vi "RSZVB Trace Response Data All Data.vi"(8 "error in (no error)":errorcluster {"code" format="%.0x"}, 9 "Data Format (0)":i32(ring) items=["Unformatted", "Formatted", "Unformatted With Trace Mathematics"], 10 "Channel (Trace) (1)":i32=1, 11 "VISA session":refnum<visa-resource-name>) -> (0 "error out":errorcluster {"code" format="%.0x"}, 3 "dup VISA session":refnum<visa-resource-name>, 5 "Trace Data":dbl[](array[numeric]) format="%^.3e")   [LabVIEW 2011]
doc: "Reads the current response values of all data traces of the current test setup.\n\nRemote-control command(s):\nFORMat[:DATA] REAL ,32\nCALCulate<Chn>:DATA:DALL? FDATa | SDATa | MDATa"
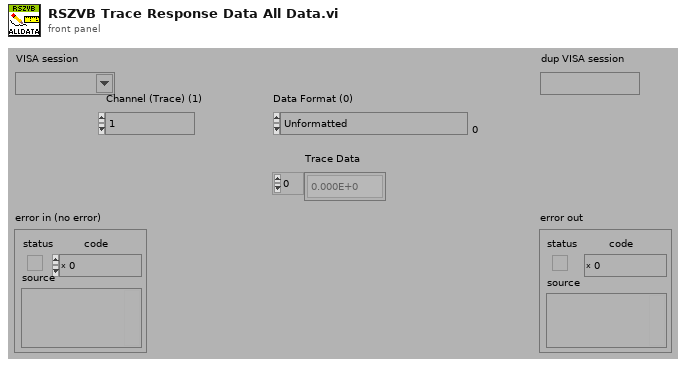
[diagram p1: front panel]
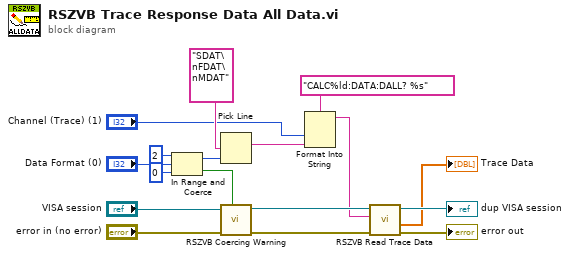
[diagram p0: block diagram]
diagram:
  n1 = In Range and Coerce(upper limit=2, x="Data Format (0)", lower limit=0) -> (coerced(x)=w11:i32, In Range?=w12:bool)
  n2 = Pick Line(multi-line string="SDAT\nFDAT\nMDAT", line index=w11) -> (output string=w7:string)  [unwired: 1 in]
  n3 = call "RSZVB Coercing Warning.vi"("In Range?"=w12, "error in (no error)"="error in (no error)", "VISA session"="VISA session") -> ("error out"=w6:errorcluster, "dup VISA session"=w5:refnum<visa-resource-name>)  [unwired: 7 in]
  n4 = Format Into String(format string="CALC%ld:DATA:DALL? %s", "Channel (Trace) (1)", w7) -> (resulting string=w4:string)  [unwired: 2 in, 1 out]
  n5 = call "RSZVB Read Trace Data.vi"("error in (no error)"=w6, "Buffer"=w4, "VISA session"=w5) -> ("error out"=→"error out":errorcluster, "Trace Data"=→"Trace Data":dbl[], "dup VISA session"=→"dup VISA session":refnum<visa-resource-name>)  [unwired: 6 in]
